vi "communicate_XYstage.vi"() -> ()   [LabVIEW 2019]
uses:
  <vilib>/Instr/_visa.llb/VISA Configure Serial Port (Instr).vi
panel:
  in  "speed?":bool
  out "concatenated string":string
  out "Array":string[][](array[string])
  out "pogress":dbl(slide) scale=0.0..1.0
  in  "write buffer":string
  out "position checking":string
  out "initial":string
  out "N try":i32
  out "done":i32
  out "total":i32
  in  "file (use dialog)":path
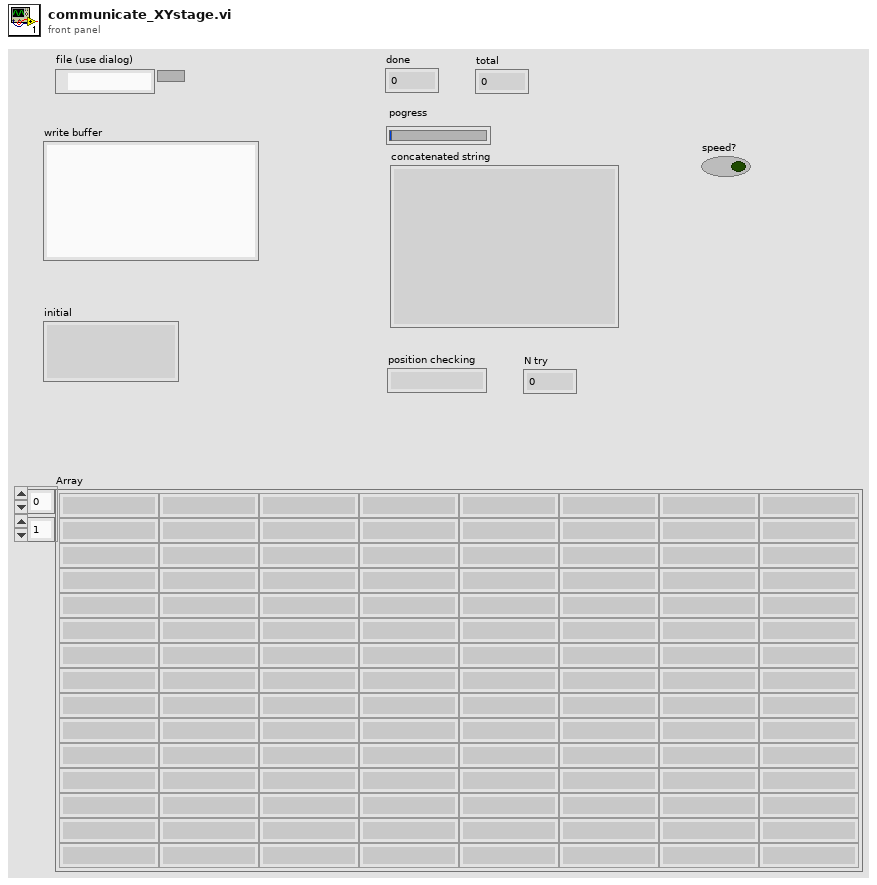
[diagram p1: front panel]
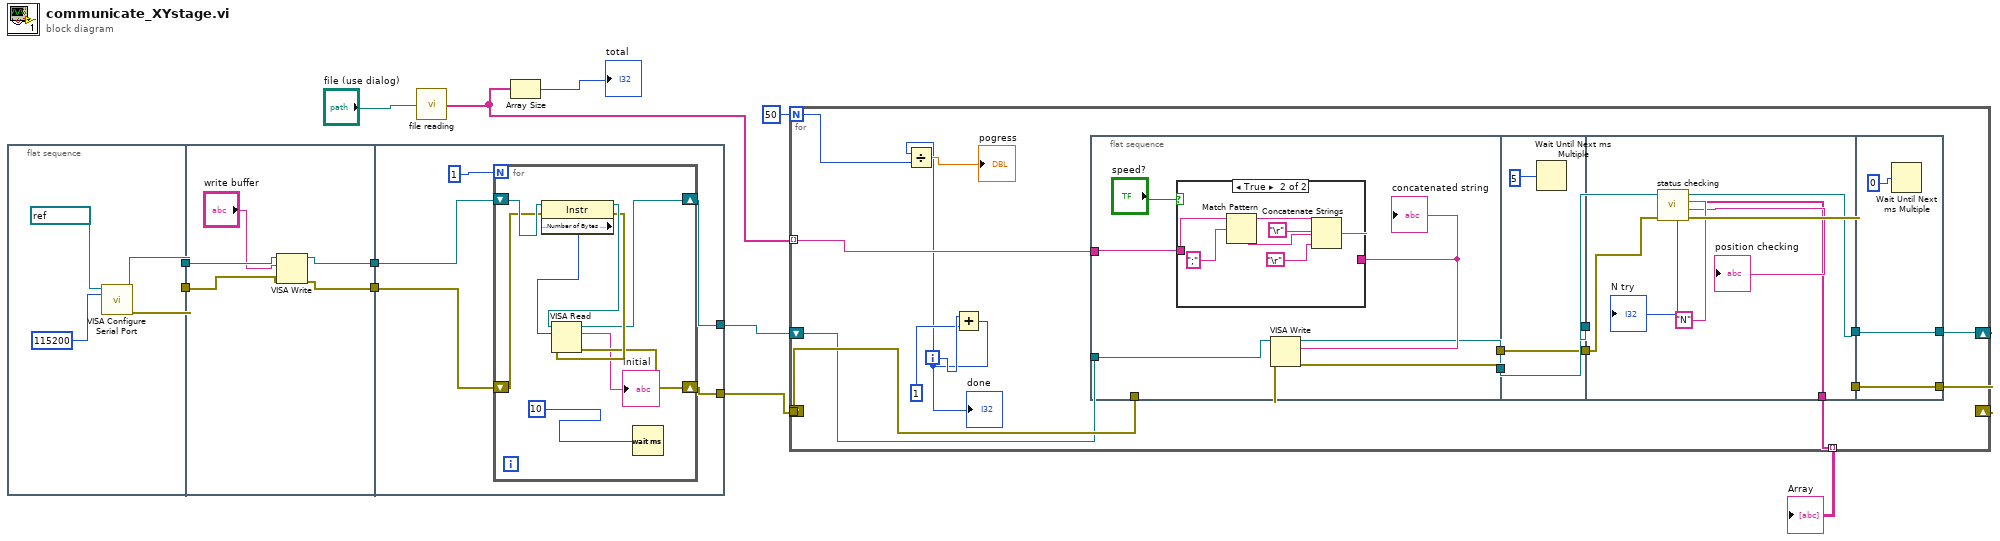
[diagram p0: block diagram]
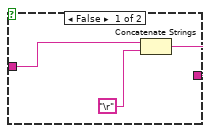
[diagram p2: hidden frame]
diagram:
  n1 = flat-sequence {
    tunnel: [w15] -> w7
    tunnel: [w14] -> w5
    tunnel: w7 -> [w20]
    tunnel: [w17] -> w6
    tunnel: w5 -> [w19]
    tunnel: [w18] -> w4
    tunnel: w6 -> [w25]
    tunnel: w4 -> [w24]
    tunnel: [w23] -> w9
    tunnel: [w22] -> w8
    frame #0 {
      n2 = call-poly "VISA Configure Serial Port"("VISA resource name"=refnum<visa-resource-name> "COM1", "baud rate (115200)"=u32 115200) -> ("VISA resource name out"=w15:refnum<visa-resource-name>, "error out"=w14:errorcluster)  [unwired: 12 in]
    }
    frame #1 {
      n3 = VISA Write(VISA resource name=w20, write buffer="write buffer", error in (no error)=w19) -> (VISA resource name out=w17:refnum<visa-resource-name>, error out=w18:errorcluster)  [unwired: 1 out]
    }
    frame #2 {
      n4 = for {
        N: 1 -> [_]
        shift-right: [w29] -> w23
        shift-left: w25 -> [w34]
        shift-right: [w28] -> w22
        shift-left: w24 -> [w33]
        n5 = property class="Instr"(reference=w34, error in=w33) -> (reference out=w32:refnum<visa-resource-name>, error out=w31:errorcluster, "Serial Settings:Number of Bytes at Serial Port"=w30:u32)
        n6 = VISA Read(VISA resource name=w32, byte count=w30, error in (no error)=w31) -> (VISA resource name out=w29:refnum<visa-resource-name>, read buffer=→"initial":string, error out=w28:errorcluster)  [unwired: 1 out]
        n7 = Wait (ms)(milliseconds to wait=u32 10) -> ()  [unwired: 1 out]
      }
    }
  }
  n8 = call "file reading.vi"("file (use dialog)"="file (use dialog)") -> ("text"=w10:string[])
  n9 = Array Size(array=w10) -> (size(s)=→"total":i32)
  n10 = for {
    N: 50 -> [w47]
    tunnel: w10 -> [w51] mode=indexing
    shift-right: [w48] -> _
    shift-left: w9 -> [w49]
    tunnel: w8 -> [w50]
    shift-right: [w36] -> _
    shift-left: _ -> [_]
    tunnel: [w35] -> w1 mode=indexing
    i -> [w41]
    n11 = Add(x=w41, y=1) -> (x+y=w39:i32)
    "done" <- w39
    n12 = Divide(x=w39, y=w47) -> (x/y=→"pogress":dbl)
    n13 = flat-sequence {
      tunnel: w49 -> [w53]
      tunnel: w50 -> [w52]
      tunnel: w51 -> [w55]
      tunnel: [w54] -> w45
      tunnel: [w58] -> w42
      tunnel: w45 -> [w71]
      tunnel: [w71] -> w44
      tunnel: [w70] -> w43
      tunnel: w42 -> [w70]
      tunnel: w44 -> [w73]
      tunnel: w43 -> [w74]
      tunnel: [w79] -> w38
      tunnel: [w75] -> w37
      tunnel: [w72] -> w35
      tunnel: [w81] -> w48
      tunnel: [w82] -> w36
      tunnel: w38 -> [w82]
      tunnel: w37 -> [w81]
      frame #0 {
        n14 = case shown="True" "speed?" {
          tunnel: [w60 w63] -> w56
          tunnel: w55 -> [w59 w62]
          frame False {
            n15 = Concatenate Strings(w59, "\r") -> (w60:string)
          }
          frame True {
            n16 = Match Pattern(string=w62, regular expression=";") -> (before substring=w66:string, after substring=w65:string)  [unwired: 1 in, 2 out]
            n17 = Concatenate Strings(w66, "\r", w65, "\r") -> (w63:string)
          }
        }
        "concatenated string" <- w56
        n18 = VISA Write(VISA resource name=w53, write buffer=w56, error in (no error)=w52) -> (VISA resource name out=w54:refnum<visa-resource-name>, error out=w58:errorcluster)  [unwired: 1 out]
      }
      frame #1 {
        n19 = Wait Until Next ms Multiple(millisecond multiple=u32 5 ("milliseconds to wait")) -> ()  [unwired: 1 out]
      }
      frame #2 {
        n20 = call "status checking.vi"("error in (no error)"=w74, "search string"="N", "VISA Refnum in"=w73) -> ("error out"=w79:errorcluster, "position checking"=→"position checking":string, "Array"=w72:string[], "VISA Refnum out"=w75:refnum<visa-resource-name>, "N try"=→"N try":i32)  [unwired: 4 in]
      }
      frame #3 {
        n21 = Wait Until Next ms Multiple(millisecond multiple=u32 0) -> ()  [unwired: 1 out]
      }
    }
  }
  "Array" <- w1
